vi "Camera Angle Calc.vi"(1 "Front Camera In":T1) -> (0 "Front Camera Out":T1)   [LabVIEW 2013]
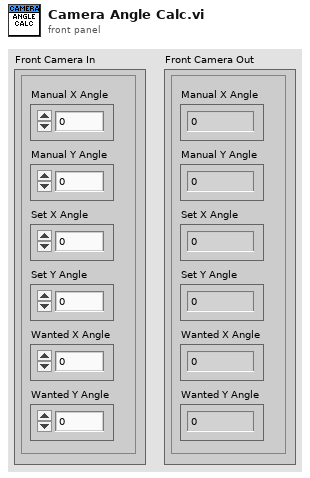
[diagram p1: front panel]
types:
  T1 = cluster{"Manual X Angle":dbl, "Manual Y Angle ":dbl, "Set X Angle":dbl, "Set Y Angle ":dbl, "Wanted X Angle":dbl, "Wanted Y Angle  ":dbl}
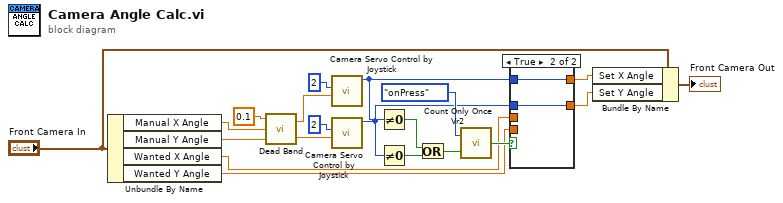
[diagram p0: block diagram]
diagram:
  n1 = Unbundle By Name("Front Camera In") -> ("Manual X Angle"=w16:dbl, "Manual Y Angle"=w15:dbl, "Wanted X Angle"=w3:dbl, "Wanted Y Angle"=w2:dbl)
  n2 = call "Dead Band.vi"("Axis 2 In"=w15, "Axis 1 In"=w16, "Dead Band"=0.1) -> ("Axis 2 Out"=w13:dbl, "Axis 1 Out"=w14:dbl)
  n3 = call "Camera Servo Control by Joystick.vi"("axis control"=w14, "max jump angle"=2) -> ("angle set"=w6:i32)  [unwired: 9 in]
  n4 = call "Camera Servo Control by Joystick.vi"("axis control"=w13, "max jump angle"=2) -> ("angle set"=w4:i32)  [unwired: 9 in]
  n5 = Not Equal To 0?(x=w6) -> (x != 0?=w12:bool)
  n6 = Not Equal To 0?(x=w4) -> (x != 0?=w11:bool)
  n7 = Or(x=w12, y=w11) -> (x .or. y?=w9:bool)
  n8 = call "Count Only Once Vr2.vi"("InValue"=w9, "Action"=enum16{"onPress", "onRelease", "Both"}."onPress") -> ("Result"=w8:bool)
  n9 = case shown="True" w8 {
    tunnel: [w22 w24] -> w7
    tunnel: w6 -> [_ w24]
    tunnel: [w21 w23] -> w5
    tunnel: w4 -> [_ w23]
    tunnel: w3 -> [w22 _]
    tunnel: w2 -> [w21 _]
    frame False {
    }
    frame True {
    }
  }
  n10 = Bundle By Name(cluster="Front Camera In", "Set X Angle"=w7, "Set Y Angle"=w5) -> (→"Front Camera Out":T1)
